vi "GDSProject_GuessFolderPath.vi"(1 "ProjectItem":refnum<vi>, 5 "error in (no error)":errorcluster) -> (15 "Path":path, 16 "FoldersToCreate":string, 17 "FolderScopes":T1(array[ring]), 19 "error out":errorcluster)   [LabVIEW 2020]
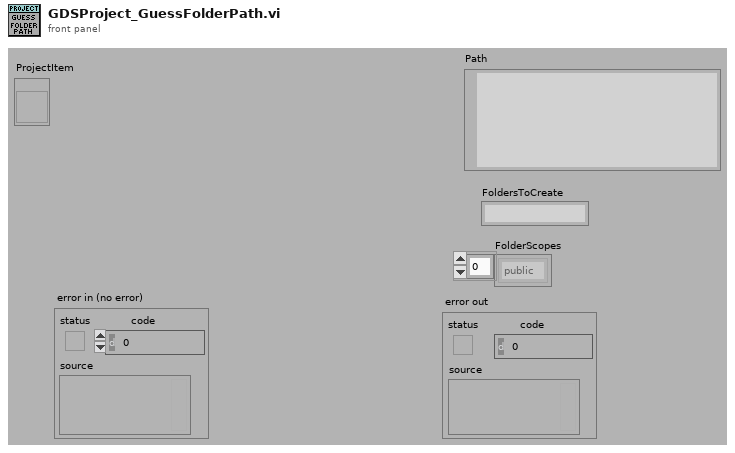
[diagram p1: front panel]
types:
  T1 = enum32{"invalid scope", "public", "private", "protected", "community"}[]
  T2 = enum32{"invalid scope", "public", "private", "protected", "community"}
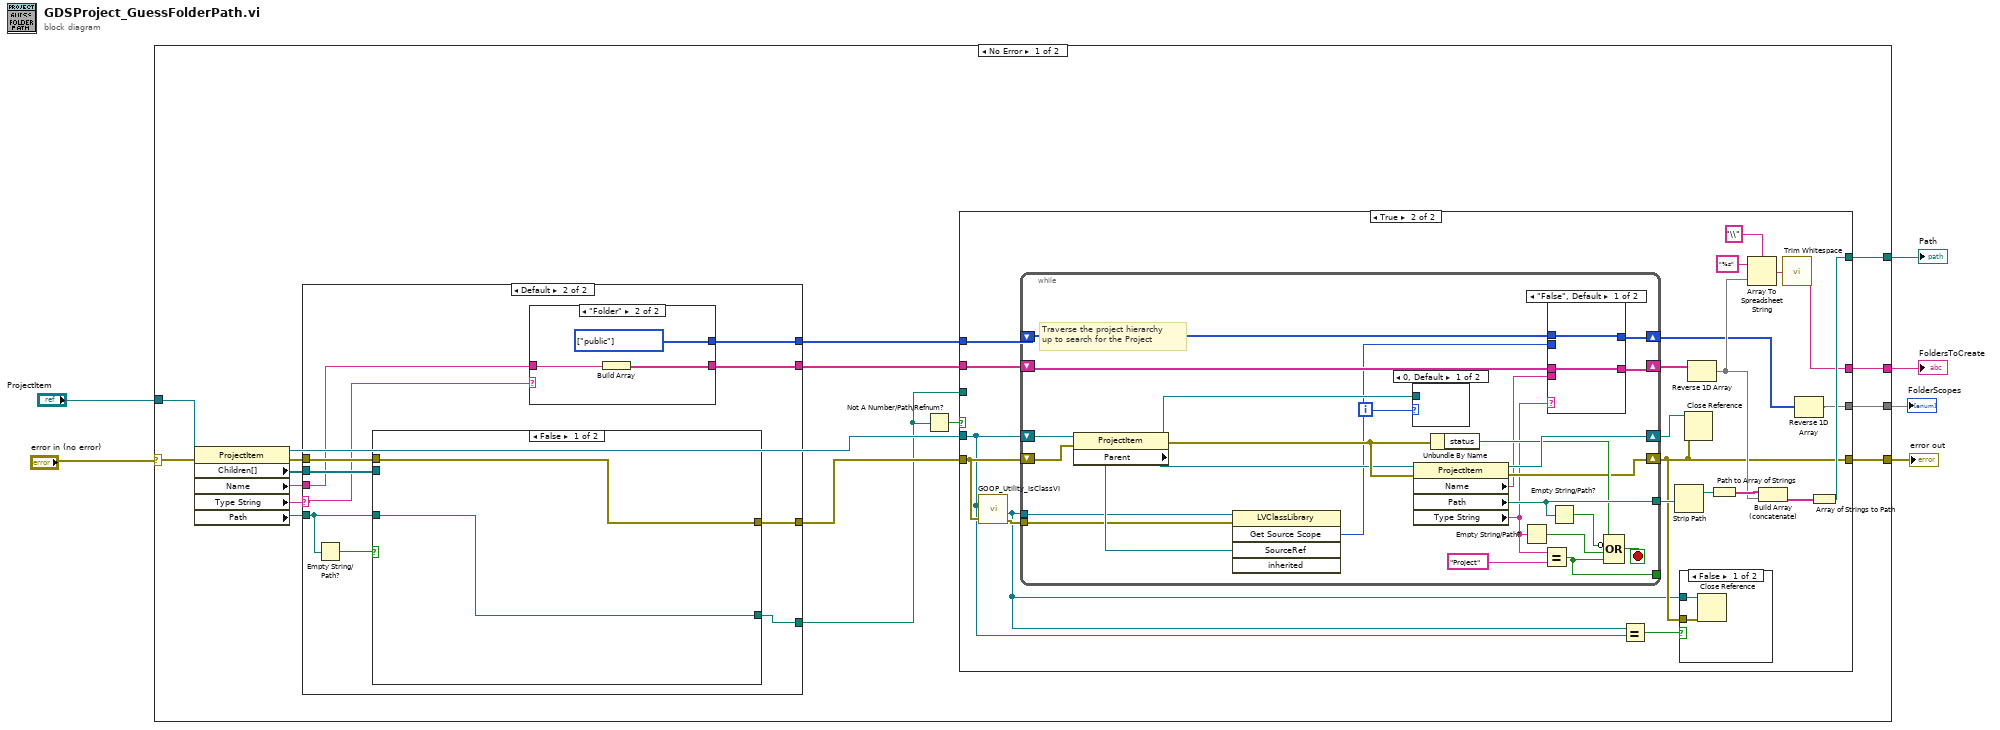
[diagram p0: block diagram]
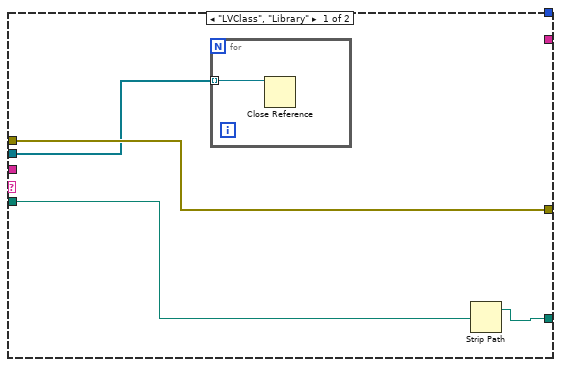
[diagram p2: hidden frame]
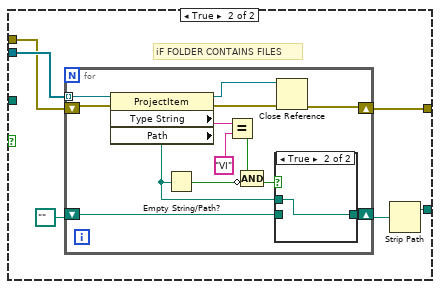
[diagram p3: hidden frame]
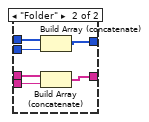
[diagram p8: hidden frame]
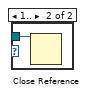
[diagram p9: hidden frame]
diagram:
  n1 = case shown="No Error" "error in (no error)" {
    selector: "error in (no error)" -> [w20 w124]
    tunnel: [w21 w124] -> w5
    tunnel: "ProjectItem" -> [w19 _]
    tunnel: [w22 _] -> w4
    tunnel: [w14 _] -> w3
    tunnel: [w12 _] -> w2
    frame No Error {
      n2 = property class="ProjectItem"(reference=w19, error in=w20) -> (reference out=w10:refnum<vi>, error out=w17:errorcluster, "Children[]"=w18:refnum<vi>[], "Name"=w16:string, "Type String"=w9:string, "Path"=w8:path)
      n3 = case shown="Default" w9 {
        selector: w9 -> [_ w32]
        tunnel: w18 -> [w26 w38]
        tunnel: [w24 w31] -> w7
        tunnel: w17 -> [w27 w37]
        tunnel: w16 -> [_ w36]
        tunnel: [_ w35] -> w15
        tunnel: [_ w34] -> w13
        tunnel: [w27 w33] -> w11
        tunnel: w8 -> [w25 w29]
        frame "LVClass", "Library" {
          n4 = for {
            tunnel: w26 -> [w28] mode=indexing
            n5 = Close Reference(reference=w28) -> ()  [unwired: 1 in, 1 out]
          }
          n6 = Strip Path(path=w25) -> (stripped path=w24:path)  [unwired: 1 out]
        }
        frame Default {
          n7 = Empty String/Path?(string/path=w29) -> (empty?=w30:bool)
          n8 = case shown="False" w30 {
            tunnel: w38 -> [_ w46]
            tunnel: w37 -> [w39 w44]
            tunnel: [w39 w43] -> w33
            tunnel: [w40 w41] -> w31
            tunnel: w29 -> [w40 _]
            frame False {
            }
            frame True {
              # "iF FOLDER CONTAINS FILES"
              n9 = for {
                shift-right: [w53] -> w43
                shift-left: w44 -> [w59]
                tunnel: w46 -> [w58] mode=indexing
                shift-right: [w56] -> w42
                shift-left: path "" ("Path") -> [w57]
                n10 = property class="ProjectItem"(reference=w58, error in=w59) -> (reference out=w55:refnum<vi>, error out=w54:errorcluster, "Type String"=w48:string, "Path"=w52:path)
                n11 = Empty String/Path?(string/path=w52) -> (empty?=w51:bool)
                n12 = Equal?(x=w48, y="VI") -> (x = y?=w49:bool)
                n13 = Compound Arithmetic op=AND(w49, invert w51) -> (w50:bool)
                n14 = case shown="True" w50 {
                  tunnel: w57 -> [w60 _]
                  tunnel: [w60 w61] -> w56
                  tunnel: w52 -> [_ w61]
                  frame False {
                  }
                  frame True {
                  }
                }
                n15 = Close Reference(reference=w55, error in (no error)=w54) -> (error out=w53:errorcluster)
              }
              n16 = Strip Path(path=w42) -> (stripped path=w41:path)  [unwired: 1 out]
            }
          }
          n17 = case shown="\"Folder\"" w32 {
            tunnel: w36 -> [_ w64]
            tunnel: [_ w63] -> w35
            tunnel: [_ w62] -> w34
            frame Default {
            }
            frame "Folder" {
              w62 = T1 [enum."public"] items=["invalid scope", "public", "private", "protected", "community"]
              n18 = Build Array(w64) -> (w63:string[])
            }
          }
        }
      }
      n19 = Not A Number/Path/Refnum?(number/path/refnum=w7) -> (NaN/Path/Refnum?=w23:bool)
      n20 = case shown="True" w23 {
        tunnel: w11 -> [w65 w71]
        tunnel: w10 -> [_ w69]
        tunnel: [w66 w87] -> w22
        tunnel: w7 -> [w66 _]
        tunnel: [w65 w72] -> w21
        tunnel: w15 -> [_ w82]
        tunnel: [_ w75] -> w14
        tunnel: w13 -> [_ w77]
        tunnel: [_ w73] -> w12
        frame False {
        }
        frame True {
          n21 = call <resource>:"GOOP_Utility_IsClassVI.vi"("error in (no error)"=w71, "ProjectItem"=w69) -> ("error out"=w70:errorcluster, "ClassItem(If Found)"=w68:refnum<vi>)  [unwired: 5 in, 3 out]
          n22 = while {
            shift-right: [w113] -> w83
            shift-left: w69 -> [w114]
            tunnel: [w106] -> w85
            tunnel: [w107] -> _
            shift-right: [w102] -> w72
            shift-left: w71 -> [w96]
            shift-right: [w99] -> w81
            shift-left: w82 -> [w100]
            shift-right: [w94] -> w74
            shift-left: w77 -> [w93]
            tunnel: w68 -> [w92]
            tunnel: w70 -> [w91]
            i -> [w109]
            stop <- w112 stop-if-true
            # "Traverse the project hierarchy\nup to search for the Project"
            n23 = property class="ProjectItem"(reference=w114, error in=w96) -> (reference out=w110:refnum<vi>, error out=w103:errorcluster, "Parent"=w97:refnum<vi>)
            n24 = invoke class="LVClassLibrary" method="Get Source Scope"(reference=w92, error in=w91, "SourceRef"=w97) -> ("GetSourceScope"=w95:T2)  [unwired: 2 in, 4 out]
            n25 = case shown="0, Default" w109 {
              tunnel: w110 -> [_ w123]
              frame 0, Default {
              }
              frame 1.. {
                n26 = Close Reference(reference=w123) -> ()  [unwired: 1 in, 1 out]
              }
            }
            n27 = property class="ProjectItem"(reference=w97, error in=w103) -> (reference out=w113:refnum<vi>, error out=w102:errorcluster, "Name"=w98:string, "Path"=w106:path, "Type String"=w101:string)
            n28 = Unbundle By Name(w103) -> ("status"=w105:bool)
            n29 = Empty String/Path?(string/path=w101) -> (empty?=w108:bool)
            n30 = Equal?(x=w101, y="Project") -> (x = y?=w107:bool)
            n31 = case shown="\"False\", Default" w101 {
              tunnel: w100 -> [w116 w122]
              tunnel: [w116 w121] -> w99
              tunnel: w98 -> [_ w120]
              tunnel: w95 -> [_ w119]
              tunnel: [w115 w118] -> w94
              tunnel: w93 -> [w115 w117]
              frame "False", Default {
              }
              frame "Folder" {
                n32 = Build Array (concatenate)(w117, w119) -> (w118:T1)
                n33 = Build Array (concatenate)(w122, w120) -> (w121:string[])
              }
            }
            n34 = Empty String/Path?(string/path=w106) -> (empty?=w104:bool)
            n35 = Compound Arithmetic op=OR(w105, invert w104, w108, w107) -> (w112:bool)
          }
          n36 = Equal?(x=w68, y=w69) -> (x = y?=w67:bool)
          n37 = Strip Path(path=w85) -> (stripped path=w84:path)  [unwired: 1 out]
          n38 = case shown="False" w67 {
            tunnel: w72 -> [w90 _]
            tunnel: w68 -> [w89 _]
            frame False {
              n39 = Close Reference(reference=w89, error in (no error)=w90) -> ()  [unwired: 1 out]
            }
            frame True {
            }
          }
          n40 = Close Reference(reference=w83, error in (no error)=w72) -> ()  [unwired: 1 out]
          n41 = Reverse 1D Array(array=w81) -> (reversed array=w76:string[])
          n42 = Path to Array of Strings(0:w84) -> (2:w88:string[])  [unwired: 1 out]
          n43 = Array To Spreadsheet String(delimiter (Tab)="\\", array=w76, 3:"%s" ("format string")) -> (spreadsheet string=w78:string)
          n44 = Build Array (concatenate)(w88, w76) -> (w86:string[])
          n45 = call <vilib>:"Trim Whitespace.vi"("string"=w78) -> ("trimmed string"=w75:string)  [unwired: 1 in]
          n46 = Reverse 1D Array(array=w74) -> (reversed array=w73:T1)
          n47 = Array of Strings to Path(0:w86) -> (2:w87:path)  [unwired: 1 in]
        }
      }
    }
    frame Error {
    }
  }
  "error out" <- w5
  "Path" <- w4
  "FoldersToCreate" <- w3
  "FolderScopes" <- w2
